vi "Get_pulses.vi"(2 "Offset":dbl(slide) scale=-1.0..1.0, 6 "Frequency":dbl, 7 "Locations":dbl[](array[numeric]), 9 "points_to_half_max":dbl, 10 "waveform in":waveform(dbl), 11 "Number of sines":dbl) -> (3 "Pulses":waveform(dbl)[](array[waveform]))   [LabVIEW 2015]
uses:
  <vilib>/Waveform/WDTOps.llb/WDT Get Waveform Subset DBL.vi
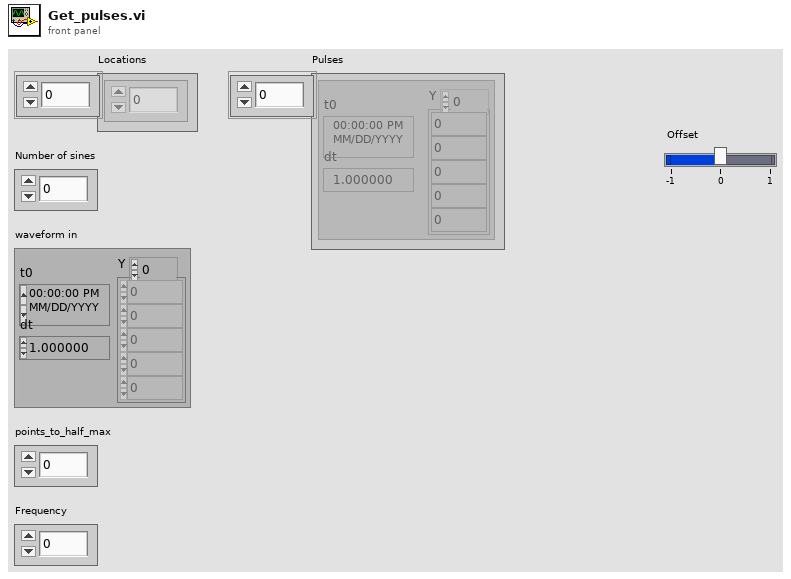
[diagram p1: front panel]
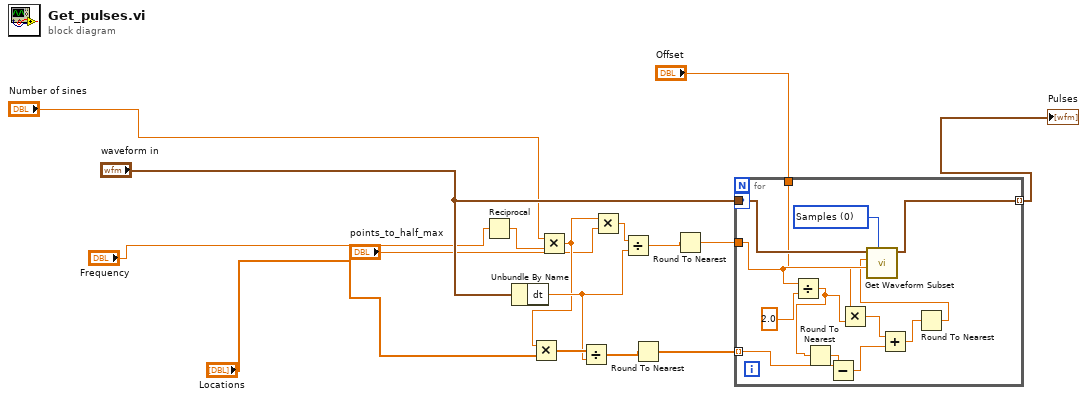
[diagram p0: block diagram]
diagram:
  n1 = Reciprocal(x="Frequency") -> (1/x=w4:dbl)
  n2 = Unbundle By Name("waveform in") -> ("dt"=w12:dbl)
  n3 = Multiply(x="Number of sines", y=w4) -> (x*y=w10:dbl)
  n4 = Multiply(x=w10, y="Locations") -> (x*y=w13:dbl[])
  n5 = Divide(x=w13, y=w12) -> (x/y=w11:dbl[])
  n6 = Multiply(x=w10, y="points_to_half_max") -> (x*y=w6:dbl)
  n7 = Divide(x=w6, y=w12) -> (x/y=w7:dbl)
  n8 = Round To Nearest(number=w11) -> (nearest integer value=w14:dbl[])
  n9 = Round To Nearest(number=w7) -> (nearest integer value=w15:dbl)
  n10 = for {
    tunnel: w14 -> [w28] mode=indexing
    tunnel: w15 -> [w27]
    tunnel: "waveform in" -> [w29]
    tunnel: [w26] -> w16 mode=indexing
    tunnel: "Offset" -> [w20]
    workers-P: _ -> [_]
    w25 = u16 0 items=["Samples", "Relative Time"] ("start/duration format")
    n11 = Divide(x=w27, y=2.0) -> (x/y=w21:dbl)
    n12 = Round To Nearest(number=w21) -> (nearest integer value=w23:dbl)
    n13 = Subtract(x=w28, y=w23) -> (x-y=w22:dbl)
    n14 = Multiply(x=w20, y=w21) -> (x*y=w19:dbl)
    n15 = Add(x=w19, y=w22) -> (x+y=w18:dbl)
    n16 = Round To Nearest(number=w18) -> (nearest integer value=w17:dbl)
    n17 = call-poly <vilib>:"Get Waveform Subset.vi"("start/duration format"=w25, "duration"=w27, "start samples/time"=w17, "waveform in"=w29) -> ("waveform out"=w26:waveform(dbl))  [unwired: 2 in, 3 out]
  }
  "Pulses" <- w16
